vi "FGV_MacroRules.vi"() -> ()   [LabVIEW 2012]
doc: "SciScan 1.2 160622"
panel:
  in  "Argument Type":enum16{"Numeric", "String", "Path"}(ring)
  out "Argument Name":string
  out "Number of Arguments":dbl
  out "ArgumentRule":T1(ring)
  in  "Command":string
  in  "FGV_MacroRules_Command":enum16{"Initialize", "GetCommandDetail"}(ring)
  out "Error Out":errorcluster
  in  "Error In":errorcluster
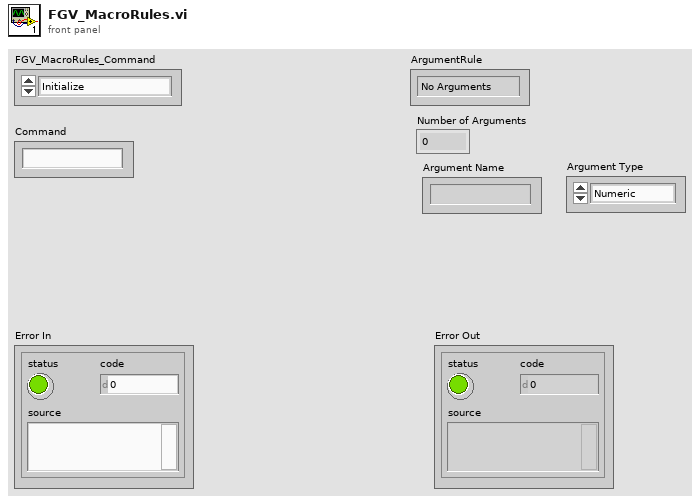
[diagram p1: front panel]
types:
  T1 = enum16{"No Arguments", "Flexible number of args", "Exact no of Args"}
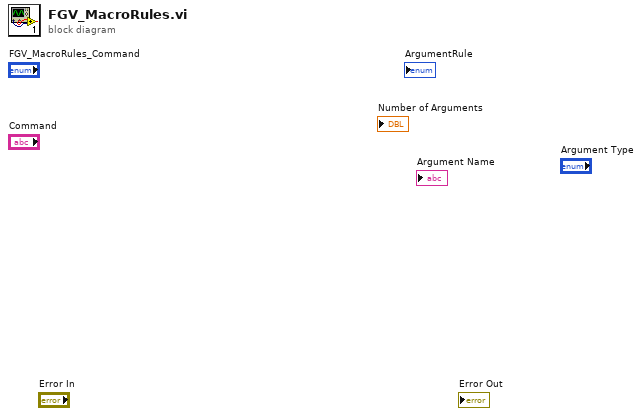
[diagram p0: block diagram]
diagram:
